vi "temperatura_vode.vi"(8 "Heating":bool) -> (2 "Temperature":dbl)   [LabVIEW 2019]
doc: "This VI simulates the heating of water in the Coffee machine water reservoir. The rate of heating is chosen at random, so the water has 50% chance of heating up to 85 C in 10 seconds or less.\nThe heating starts when the Boolean input \"Heating\" is set to True.\nChanging the Boolean input \"Heating\" to False resets the water temperature to 25 C.\nThe output is the temperature in degrees Celsius."
uses:
  <vilib>/express/express arith-compare/Formula/XNode/ExpressFormulaBlockNode.xnode
panel:
  out "x-y":u32
  out "start time":u32
  out "Heating rate":dbl
  in  "First call":bool
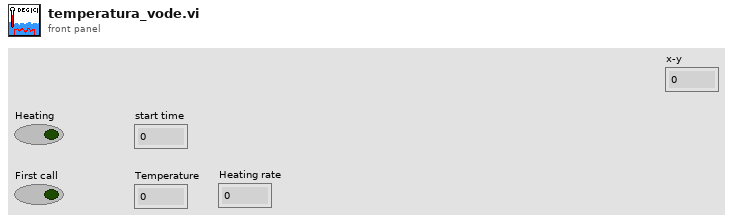
[diagram p1: front panel]
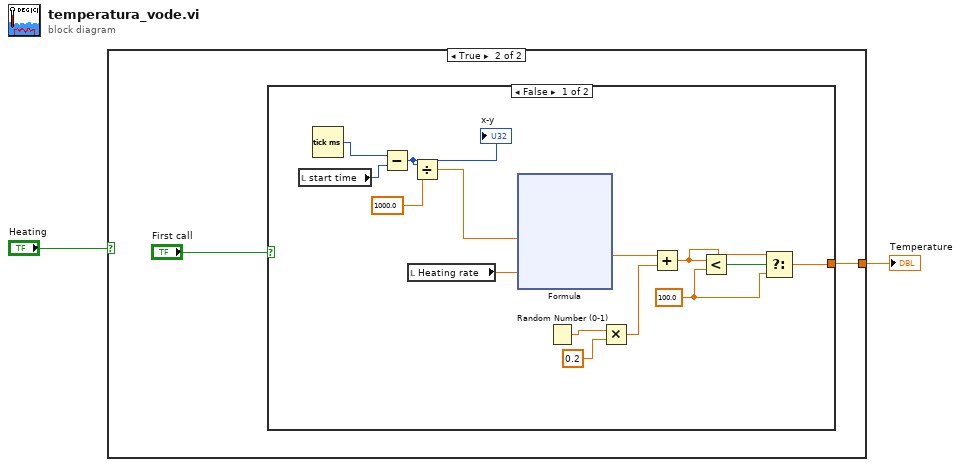
[diagram p0: block diagram]
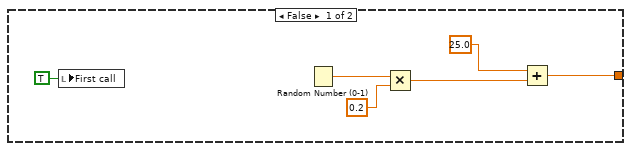
[diagram p2: hidden frame]
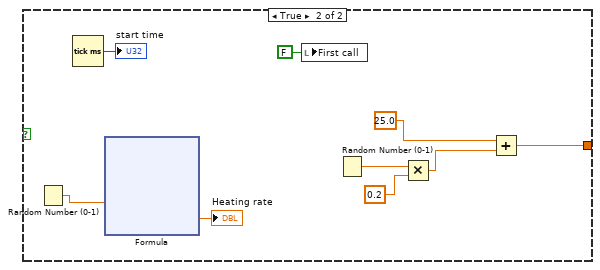
[diagram p3: hidden frame]
diagram:
  n1 = case shown="True" "Heating" {
    tunnel: [w3 w9] -> w2
    frame False {
      n2 = local write "First call"(TRUE ("First call")) -> ()
      n3 = Random Number (0-1)() -> (number: 0 to 1=w7:dbl)
      n4 = Multiply(x=w7, y=0.2) -> (x*y=w4:dbl)
      n5 = Add(x=25.0, y=w4) -> (x+y=w3:dbl)
    }
    frame True {
      n6 = case shown="False" "First call" {
        tunnel: [w12 w35] -> w9
        frame False {
          w13 = 100.0 ("f")
          n7 = local read "start time"() -> (w22:u32)
          n8 = Tick Count (ms)() -> (millisecond timer value=w23:u32)
          n9 = Subtract(x=w23, y=w22) -> (x-y=w11:u32)
          "x-y" <- w11
          n10 = local read "Heating rate"() -> (w24:dbl)
          n11 = Divide(x=w11, y=1000.0) -> (x/y=w20:dbl)
          n12 = xnode "Formula"("time"=w20, "tau"=w24) -> ("Result"=w16:dbl)  [unwired: 1 in, 1 out]
          n13 = Random Number (0-1)() -> (number: 0 to 1=w19:dbl)
          n14 = Multiply(x=w19, y=0.2) -> (x*y=w17:dbl)
          n15 = Add(x=w16, y=w17) -> (x+y=w14:dbl)
          n16 = Less?(x=w14, y=w13) -> (x < y?=w15:bool)
          n17 = Select(t=w14, s=w15, f=w13) -> (s? t:f=w12:dbl)
        }
        frame True {
          n18 = Random Number (0-1)() -> (number: 0 to 1=w43:dbl)
          n19 = Tick Count (ms)() -> (millisecond timer value=→"start time":u32)
          n20 = xnode "Formula"("rand"=w43) -> ("Result"=→"Heating rate":dbl)  [unwired: 1 in, 1 out]
          n21 = local write "First call"(FALSE ("First call")) -> ()
          n22 = Random Number (0-1)() -> (number: 0 to 1=w39:dbl)
          n23 = Multiply(x=w39, y=0.2) -> (x*y=w37:dbl)
          n24 = Add(x=25.0, y=w37) -> (x+y=w35:dbl)
        }
      }
    }
  }
  "Temperature" <- w2
